vi "nanocal -- nuclear schottky fit V7.vi"() -> ()   [LabVIEW 2021] (continued)
 -> 0.201723581349   ,  \"T\" -> 0.820000000000   ,  \"B\" -> 2.000000000000   ,  \"θ\" -> 0.000000000000   ,  \"Reoff\" -> -1142857.142857141790   ,  \"Imoff\" -> 0.000000000000   ,  \"στ1\" -> 0.016798355334   ,  \"στS\" -> 0.000164505064   ,  \"στN\" -> 0.000022903136    |>   , \n\"IDS0569_220607_RAW_cal__sam_\" ->   <|    \"ζ\" -> 0.000000000000   ,  \"τ1\" -> 0.000000000000   ,  \"τS\" -> 0.000000000000   ,  \"τN\" -> 0.000000000000   ,  \"τC\" -> 0.000000000000   ,  \"κ0\" -> 0.000000000000   ,  \"mm1\" -> 0.000000000000   ,  \"mm2\" -> 0.000000000000   ,  \"mm3\" -> 0.000000000000   ,  \"T\" -> 0.820000000000   ,  \"B\" -> 2.000000000000   ,  \"θ\" -> 0.000000000000   ,  \"Reoff\" -> 0.000000000000   ,  \"Imoff\" -> 0.000000000000   ,  \"στ1\" -> 0.000000000000   ,  \"στS\" -> 0.000000000000   ,  \"στN\" -> 0.000000000000    |>   , \n\"IDS0570_220607_RAW_cal__ref_\" ->   <|    \"ζ\" -> 0.023186603119   ,  \"τ1\" -> 0.069304039551   ,  \"τS\" -> 0.024728755203   ,  \"τN\" -> 0.000615822915   ,  \"τC\" -> 0.002362965503   ,  \"κ0\" -> 0.000000007147   ,  \"mm1\" -> 0.000049060818   ,  \"mm2\" -> 0.027208827859   ,  \"mm3\" -> 0.070341349169   ,  \"T\" -> 1.120000000000   ,  \"B\" -> 2.000000000000   ,  \"θ\" -> 0.000000000000   ,  \"Reoff\" -> -897959.183673471211   ,  \"Imoff\" -> 0.000000000000   ,  \"στ1\" -> 0.007066895477   ,  \"στS\" -> 0.000207495874   ,  \"στN\" -> 0.000024034388    |>   , \n\"IDS0570_220607_RAW_cal__sam_\" ->   <|    \"ζ\" -> 0.000000000000   ,  \"τ1\" -> 0.000000000000   ,  \"τS\" -> 0.000000000000   ,  \"τN\" -> 0.000000000000   ,  \"τC\" -> 0.000000000000   ,  \"κ0\" -> 0.000000000000   ,  \"mm1\" -> 0.000000000000   ,  \"mm2\" -> 0.000000000000   ,  \"mm3\" -> 0.000000000000   ,  \"T\" -> 1.120000000000   ,  \"B\" -> 2.000000000000   ,  \"θ\" -> 0.000000000000   ,  \"Reoff\" -> 0.000000000000   ,  \"Imoff\" -> 0.000000000000   ,  \"στ1\" -> 0.000000000000   ,  \"στS\" -> 0.000000000000   ,  \"στN\" -> 0.000000000000    |>   , \n\"IDS0571_220607_RAW_cal__ref_\" ->   <|    \"ζ\" -> 0.015770363513   ,  \"τ1\" -> 0.071971798635   ,  \"τS\" -> 0.047933574846   ,  \"τN\" -> 0.000365152941   ,  \"τC\" -> 0.002700044906   ,  \"κ0\" -> 0.000000012652   ,  \"mm1\" -> 0.000039747850   ,  \"mm2\" -> 0.050478715429   ,  \"mm3\" -> 0.073213796543   ,  \"T\" -> 1.900000000000   ,  \"B\" -> 2.000000000000   ,  \"θ\" -> 0.000000000000   ,  \"Reoff\" -> -285714.285714287310   ,  \"Imoff\" -> 0.000000000000   ,  \"στ1\" -> 0.006975803229   ,  \"στS\" -> 0.000442024056   ,  \"στN\" -> 0.000016462134    |>   , \n\"IDS0571_220607_RAW_cal__sam_\" ->   <|    \"ζ\" -> 0.000000000000   ,  \"τ1\" -> 0.000000000000   ,  \"τS\" -> 0.000000000000   ,  \"τN\" -> 0.000000000000   ,  \"τC\" -> 0.000000000000   ,  \"κ0\" -> 0.000000000000   ,  \"mm1\" -> 0.000000000000   ,  \"mm2\" -> 0.000000000000   ,  \"mm3\" -> 0.000000000000   ,  \"T\" -> 1.900000000000   ,  \"B\" -> 2.000000000000   ,  \"θ\" -> 0.000000000000   ,  \"Reoff\" -> 0.000000000000   ,  \"Imoff\" -> 0.000000000000   ,  \"στ1\" -> 0.000000000000   ,  \"στS\" -> 0.000000000000   ,  \"στN\" -> 0.000000000000    |>   , \n\"IDS0572_220607_RAW_cal__ref_\" ->   <|    \"ζ\" -> 0.018018584104   ,  \"τ1\" -> 0.047661155544   ,  \"τS\" -> 0.013484677326   ,  \"τN\" -> 0.000256030731   ,  \"τC\" -> 0.002573709531   ,  \"κ0\" -> 0.000000016044   ,  \"mm1\" -> 0.000038452225   ,  \"mm2\" -> 0.016129638273   ,  \"mm3\" -> 0.048055070739   ,  \"T\" -> 2.300000000000   ,  \"B\" -> 2.000000000000   ,  \"θ\" -> 0.000000000000   ,  \"Reoff\" -> -285714.285714287310   ,  \"Imoff\" -> 0.000000000000   ,  \"στ1\" -> 0.009039480993   ,  \"στS\" -> 0.000292801167   ,  \"στN\" -> 0.000013350378    |>   , \n\"IDS0572_220607_RAW_cal__sam_\" ->   <|    \"ζ\" -> 0.000000000000   ,  \"τ1\" -> 0.000000000000   ,  \"τS\" -> 0.000000000000   ,  \"τN\" -> 0.000000000000   ,  \"τC\" -> 0.000000000000   ,  \"κ0\" -> 0.000000000000   ,  \"mm1\" -> 0.000000000000   ,  \"mm2\" -> 0.000000000000   ,  \"mm3\" -> 0.000000000000   ,  \"T\" -> 2.300000000000   ,  \"B\" -> 2.000000000000   ,  \"θ\" -> 0.000000000000   ,  \"Reoff\" -> 0.000000000000   ,  \"Imoff\" -> 0.000000000000   ,  \"στ1\" -> 0.000000000000   ,  \"στS\" -> 0.000000000000   ,  \"στN\" -> 0.000000000000    |>   , \n\"IDS0573_220607_RAW_cal__ref_\" ->   <|    \"ζ\" -> 0.017854709230   ,  \"τ1\" -> 0.048990500372   ,  \"τS\" -> 0.009409191095   ,  \"τN\" -> 0.000133052666   ,  \"τC\" -> 0.002613702785   ,  \"κ0\" -> 0.000000022548   ,  \"mm1\" -> 0.000036125485   ,  \"mm2\" -> 0.012110331944   ,  \"mm3\" -> 0.049170363477   ,  \"T\" -> 3.100000000000   ,  \"B\" -> 2.000000000000   ,  \"θ\" -> 0.000000000000   ,  \"Reoff\" -> -163265.306122448295   ,  \"Imoff\" -> 0.000000000000   ,  \"στ1\" -> 0.003929388168   ,  \"στS\" -> 0.000082158552   ,  \"στN\" -> 0.000004662808    |>   , \n\"IDS0573_220607_RAW_cal__sam_\" ->   <|    \"ζ\" -> 0.000000000000   ,  \"τ1\" -> 0.000000000000   ,  \"τS\" -> 0.000000000000   ,  \"τN\" -> 0.000000000000   ,  \"τC\" -> 0.000000000000   ,  \"κ0\" -> 0.000000000000   ,  \"mm1\" -> 0.000000000000   ,  \"mm2\" -> 0.000000000000   ,  \"mm3\" -> 0.000000000000   ,  \"T\" -> 3.100000000000   ,  \"B\" -> 2.000000000000   ,  \"θ\" -> 0.000000000000   ,  \"Reoff\" -> 0.000000000000   ,  \"Imoff\" -> 0.000000000000   ,  \"στ1\" -> 0.000000000000   ,  \"στS\" -> 0.000000000000   ,  \"στN\" -> 0.000000000000    |>   , \n\"IDS0574_220607_RAW_cal__ref_\" ->   <|    \"ζ\" -> 0.021296069589   ,  \"τ1\" -> 0.048193111718   ,  \"τS\" -> 0.005769221839   ,  \"τN\" -> 0.000085869671   ,  \"τC\" -> 0.001966024103   ,  \"κ0\" -> 0.000000055540   ,  \"mm1\" -> 0.000030859965   ,  \"mm2\" -> 0.007810308294   ,  \"mm3\" -> 0.048297749508   ,  \"T\" -> 5.700000000000   ,  \"B\" -> 2.000000000000   ,  \"θ\" -> 0.000000000000   ,  \"Reoff\" -> -89795.918367346749   ,  \"Imoff\" -> 0.000000000000   ,  \"στ1\" -> 0.003900504752   ,  \"στS\" -> 0.000042384921   ,  \"στN\" -> 0.000002866550    |>   , \n\"IDS0574_220607_RAW_cal__sam_\" ->   <|    \"ζ\" -> 0.000000000000   ,  \"τ1\" -> 0.000000000000   ,  \"τS\" -> 0.000000000000   ,  \"τN\" -> 0.000000000000   ,  \"τC\" -> 0.000000000000   ,  \"κ0\" -> 0.000000000000   ,  \"mm1\" -> 0.000000000000   ,  \"mm2\" -> 0.000000000000   ,  \"mm3\" -> 0.000000000000   ,  \"T\" -> 5.700000000000   ,  \"B\" -> 2.000000000000   ,  \"θ\" -> 0.000000000000   ,  \"Reoff\" -> 0.000000000000   ,  \"Imoff\" -> 0.000000000000   ,  \"στ1\" -> 0.000000000000   ,  \"στS\" -> 0.000000000000   ,  \"στN\" -> 0.000000000000    |>   , \n\"IDS0578_220608_RAW_cal__ref_\" ->   <|    \"ζ\" -> 0.260580240331   ,  \"τ1\" -> 0.233392220968   ,  \"τS\" -> 0.019337528339   ,  \"τN\" -> 0.006746984129   ,  \"τC\" -> 0.000809912718   ,  \"κ0\" -> 0.000000000898   ,  \"mm1\" -> 0.000163092082   ,  \"mm2\" -> 0.024046559857   ,  \"mm3\" -> 0.242874102744   ,  \"T\" -> 0.200000000000   ,  \"B\" -> 2.000000000000   ,  \"θ\" -> 90.000000000000   ,  \"Reoff\" -> -51020408.163265287900   ,  \"Imoff\" -> 0.000000000000   ,  \"στ1\" -> 0.360874017703   ,  \"στS\" -> 0.000459944418   ,  \"στN\" -> 0.007141056200    |>   , \n\"IDS0578_220608_RAW_cal__sam_\" ->   <|    \"ζ\" -> 0.000000000000   ,  \"τ1\" -> 0.000000000000   ,  \"τS\" -> 0.000000000000   ,  \"τN\" -> 0.000000000000   ,  \"τC\" -> 0.000000000000   ,  \"κ0\" -> 0.000000000000   ,  \"mm1\" -> 0.000000000000   ,  \"mm2\" -> 0.000000000000   ,  \"mm3\" -> 0.000000000000   ,  \"T\" -> 0.200000000000   ,  \"B\" -> 2.000000000000   ,  \"θ\" -> 90.000000000000   ,  \"Reoff\" -> 0.000000000000   ,  \"Imoff\" -> 0.000000000000   ,  \"στ1\" -> 0.000000000000   ,  \"στS\" -> 0.000000000000   ,  \"στN\" -> 0.000000000000    |>   , \n\"IDS0579_220608_RAW_cal__ref_\" ->   <|    \"ζ\" -> 0.358041732305   ,  \"τ1\" -> 0.218984893341   ,  \"τS\" -> 0.022109893709   ,  \"τN\" -> 0.011578421119   ,  \"τC\" -> 0.000774433851   ,  \"κ0\" -> 0.000000000705   ,  \"mm1\" -> 0.000200343737   ,  \"mm2\" -> 0.028269791705   ,  \"mm3\" -> 0.237039329177   ,  \"T\" -> 0.170000000000   ,  \"B\" -> 2.000000000000   ,  \"θ\" -> 90.000000000000   ,  \"Reoff\" -> -83673469.387755096000   ,  \"Imoff\" -> 0.000000000000   ,  \"στ1\" -> 0.324633037067   ,  \"στS\" -> 0.000730773074   ,  \"στN\" -> 0.013143956795    |>   , \n\"IDS0579_220608_RAW_cal__sam_\" ->   <|    \"ζ\" -> 0.000000000000   ,  \"τ1\" -> 0.000000000000   ,  \"τS\" -> 0.000000000000   ,  \"τN\" -> 0.000000000000   ,  \"τC\" -> 0.000000000000   ,  \"κ0\" -> 0.000000000000   ,  \"mm1\" -> 0.000000000000   ,  \"mm2\" -> 0.000000000000   ,  \"mm3\" -> 0.000000000000   ,  \"T\" -> 0.170000000000   ,  \"B\" -> 2.000000000000   ,  \"θ\" -> 90.000000000000   ,  \"Reoff\" -> 0.000000000000   ,  \"Imoff\" -> 0.000000000000   ,  \"στ1\" -> 0.000000000000   ,  \"στS\" -> 0.000000000000   ,  \"στN\" -> 0.000000000000    |>   , \n\"IDS0580_220608_RAW_cal__ref_\" ->   <|    \"ζ\" -> 0.444194308226   ,  \"τ1\" -> 0.247703542844   ,  \"τS\" -> 0.025021615076   ,  \"τN\" -> 0.015371954390   ,  \"τC\" -> 0.000794757601   ,  \"κ0\" -> 0.000000000600   ,  \"mm1\" -> 0.000240752300   ,  \"mm2\" -> 0.033248610212   ,  \"mm3\" -> 0.273345101045   ,  \"T\" -> 0.150000000000   ,  \"B\" -> 2.000000000000   ,  \"θ\" -> 90.000000000000   ,  \"Reoff\" -> -104081632.653061211000   ,  \"Imoff\" -> 0.000000000000   ,  \"στ1\" -> 0.811876218659   ,  \"στS\" -> 0.001521304973   ,  \"στN\" -> 0.040822562310    |>   , \n\"IDS0580_220608_RAW_cal__sam_\" ->   <|    \"ζ\" -> 0.000000000000   ,  \"τ1\" -> 0.000000000000   ,  \"τS\" -> 0.000000000000   ,  \"τN\" -> 0.000000000000   ,  \"τC\" -> 0.000000000000   ,  \"κ0\" -> 0.000000000000   ,  \"mm1\" -> 0.000000000000   ,  \"mm2\" -> 0.000000000000   ,  \"mm3\" -> 0.000000000000   ,  \"T\" -> 0.150000000000   ,  \"B\" -> 2.000000000000   ,  \"θ\" -> 90.000000000000   ,  \"Reoff\" -> 0.000000000000   ,  \"Imoff\" -> 0.000000000000   ,  \"στ1\" -> 0.000000000000   ,  \"στS\" -> 0.000000000000   ,  \"στN\" -> 0.000000000000    |>   , \n\"IDS0581_220608_RAW_cal__ref_\" ->   <|    \"ζ\" -> 0.686806962981   ,  \"τ1\" -> 0.191964510357   ,  \"τS\" -> 0.031477597051   ,  \"τN\" -> 0.029789944795   ,  \"τC\" -> 0.000797477821   ,  \"κ0\" -> 0.000000000433   ,  \"mm1\" -> 0.000321816656   ,  \"mm2\" -> 0.040244297441   ,  \"mm3\" -> 0.255542390272   ,  \"T\" -> 0.120000000000   ,  \"B\" -> 2.000000000000   ,  \"θ\" -> 90.000000000000   ,  \"Reoff\" -> -218367346.938775510000   ,  \"Imoff\" -> 0.000000000000   ,  \"στ1\" -> 0.248597488998   ,  \"στS\" -> 0.002831181242   ,  \"στN\" -> 0.031806706752    |>   , \n\"IDS0581_220608_RAW_cal__sam_\" ->   <|    \"ζ\" -> 0.000000000000   ,  \"τ1\" -> 0.000000000000   ,  \"τS\" -> 0.000000000000   ,  \"τN\" -> 0.000000000000   ,  \"τC\" -> 0.000000000000   ,  \"κ0\" -> 0.000000000000   ,  \"mm1\" -> 0.000000000000   ,  \"mm2\" -> 0.000000000000   ,  \"mm3\" -> 0.000000000000   ,  \"T\" -> 0.120000000000   ,  \"B\" -> 2.000000000000   ,  \"θ\" -> 90.000000000000   ,  \"Reoff\" -> 0.000000000000   ,  \"Imoff\" -> 0.000000000000   ,  \"στ1\" -> 0.000000000000   ,  \"στS\" -> 0.000000000000   ,  \"στN\" -> 0.000000000000    |>   , \n\"IDS0582_220608_RAW_cal__ref_\" ->   <|    \"ζ\" -> 0.166369563634   ,  \"τ1\" -> 0.241506341921   ,  \"τS\" -> 0.016551953229   ,  \"τN\" -> 0.004476656392   ,  \"τC\" -> 0.000955255274   ,  \"κ0\" -> 0.000000001230   ,  \"mm1\" -> 0.000130674320   ,  \"mm2\" -> 0.019667491815   ,  \"mm3\" -> 0.247190561287   ,  \"T\" -> 0.250000000000   ,  \"B\" -> 2.000000000000   ,  \"θ\" -> 90.000000000000   ,  \"Reoff\" -> -23265306.122448980800   ,  \"Imoff\" -> 0.000000000000   ,  \"στ1\" -> 0.210252832674   ,  \"στS\" -> 0.000349343663   ,  \"στN\" -> 0.005793752107    |>   , \n\"IDS0582_220608_RAW_cal__sam_\" ->   <|    \"ζ\" -> 0.000000000000   ,  \"τ1\" -> 0.000000000000   ,  \"τS\" -> 0.000000000000   ,  \"τN\" -> 0.000000000000   ,  \"τC\" -> 0.000000000000   ,  \"κ0\" -> 0.000000000000   ,  \"mm1\" -> 0.000000000000   ,  \"mm2\" -> 0.000000000000   ,  \"mm3\" -> 0.000000000000   ,  \"T\" -> 0.250000000000   ,  \"B\" -> 2.000000000000   ,  \"θ\" -> 90.000000000000   ,  \"Reoff\" -> 0.000000000000   ,  \"Imoff\" -> 0.000000000000   ,  \"στ1\" -> 0.000000000000   ,  \"στS\" -> 0.000000000000   ,  \"στN\" -> 0.000000000000    |>   , \n\"IDS0583_220608_RAW_cal__ref_\" ->   <|    \"ζ\" -> 0.118361182005   ,  \"τ1\" -> 0.150636490656   ,  \"τS\" -> 0.015529851966   ,  \"τN\" -> 0.003531374182   ,  \"τC\" -> 0.001007690492   ,  \"κ0\" -> 0.000000001529   ,  \"mm1\" -> 0.000101358307   ,  \"mm2\" -> 0.017747047219   ,  \"mm3\" -> 0.155113111027   ,  \"T\" -> 0.300000000000   ,  \"B\" -> 2.000000000000   ,  \"θ\" -> 90.000000000000   ,  \"Reoff\" -> -15102040.816326528800   ,  \"Imoff\" -> 0.000000000000   ,  \"στ1\" -> 0.078929426255   ,  \"στS\" -> 0.000167827635   ,  \"στN\" -> 0.002346663512    |>   , \n\"IDS0583_220608_RAW_cal__sam_\" ->   <|    \"ζ\" -> 0.000000000000   ,  \"τ1\" -> 0.000000000000   ,  \"τS\" -> 0.000000000000   ,  \"τN\" -> 0.000000000000   ,  \"τC\" -> 0.000000000000   ,  \"κ0\" -> 0.000000000000   ,  \"mm1\" -> 0.000000000000   ,  \"mm2\" -> 0.000000000000   ,  \"mm3\" -> 0.000000000000   ,  \"T\" -> 0.300000000000   ,  \"B\" -> 2.000000000000   ,  \"θ\" -> 90.000000000000   ,  \"Reoff\" -> 0.000000000000   ,  \"Imoff\" -> 0.000000000000   ,  \"στ1\" -> 0.000000000000   ,  \"στS\" -> 0.000000000000   ,  \"στN\" -> 0.000000000000    |>   , \n\"IDS0584_220608_RAW_cal__ref_\" ->   <|    \"ζ\" -> 0.085716797729   ,  \"τ1\" -> 0.145541921942   ,  \"τS\" -> 0.014790459938   ,  \"τN\" -> 0.003022723579   ,  \"τC\" -> 0.001204929117   ,  \"κ0\" -> 0.000000001932   ,  \"mm1\" -> 0.000088946369   ,  \"mm2\" -> 0.016747642578   ,  \"mm3\" -> 0.149250334678   ,  \"T\" -> 0.360000000000   ,  \"B\" -> 2.000000000000   ,  \"θ\" -> 90.000000000000   ,  \"Reoff\" -> -8571428.571428582080   ,  \"Imoff\" -> 0.000000000000   ,  \"στ1\" -> 0.049017314235   ,  \"στS\" -> 0.000077215540   ,  \"στN\" -> 0.000273627633    |>   , \n\"IDS0584_220608_RAW_cal__sam_\" ->   <|    \"ζ\" -> 0.000000000000   ,  \"τ1\" -> 0.000000000000   ,  \"τS\" -> 0.000000000000   ,  \"τN\" -> 0.000000000000   ,  \"τC\" -> 0.000000000000   ,  \"κ0\" -> 0.000000000000   ,  \"mm1\" -> 0.000000000000   ,  \"mm2\" -> 0.000000000000   ,  \"mm3\" -> 0.000000000000   ,  \"T\" -> 0.360000000000   ,  \"B\" -> 2.000000000000   ,  \"θ\" -> 90.000000000000   ,  \"Reoff\" -> 0.000000000000   ,  \"Imoff\" -> 0.000000000000   ,  \"στ1\" -> 0.000000000000   ,  \"στS\" -> 0.000000000000   ,  \"στN\" -> 0.000000000000    |>   , \n\"IDS0585_220608_RAW_cal__ref_\" ->   <|    \"ζ\" -> 0.064153972834   ,  \"τ1\" -> 0.145990399088   ,  \"τS\" -> 0.014755700071   ,  \"τN\" -> 0.002470459255   ,  \"τC\" -> 0.001390626850   ,  \"κ0\" -> 0.000000002341   ,  \"mm1\" -> 0.000077364865   ,  \"mm2\" -> 0.016676693112   ,  \"mm3\" -> 0.148958253844   ,  \"T\" -> 0.420000000000   ,  \"B\" -> 2.000000000000   ,  \"θ\" -> 90.000000000000   ,  \"Reoff\" -> -4530612.244897958820   ,  \"Imoff\" -> 0.000000000000   ,  \"στ1\" -> 0.010117026609   ,  \"στS\" -> 0.000141538965   ,  \"στN\" -> 0.000077781764    |>   , \n\"IDS0585_220608_RAW_cal__sam_\" ->   <|    \"ζ\" -> 0.000000000000   ,  \"τ1\" -> 0.000000000000   ,  \"τS\" -> 0.000000000000   ,  \"τN\" -> 0.000000000000   ,  \"τC\" -> 0.000000000000   ,  \"κ0\" -> 0.000000000000   ,  \"mm1\" -> 0.000000000000   ,  \"mm2\" -> 0.000000000000   ,  \"mm3\" -> 0.000000000000   ,  \"T\" -> 0.420000000000   ,  \"B\" -> 2.000000000000   ,  \"θ\" -> 90.000000000000   ,  \"Reoff\" -> 0.000000000000   ,  \"Imoff\" -> 0.000000000000   ,  \"στ1\" -> 0.000000000000   ,  \"στS\" -> 0.000000000000   ,  \"στN\" -> 0.000000000000    |>   , \n\"IDS0586_220608_RAW_cal__ref_\" ->   <|    \"ζ\" -> 0.050400440296   ,  \"τ1\" -> 0.120007371635   ,  \"τS\" -> 0.015618683096   ,  \"τN\" -> 0.001956039129   ,  \"τC\" -> 0.001501517777   ,  \"κ0\" -> 0.000000002996   ,  \"mm1\" -> 0.000066249745   ,  \"mm2\" -> 0.017490709551   ,  \"mm3\" -> 0.122412426079   ,  \"T\" -> 0.520000000000   ,  \"B\" -> 2.000000000000   ,  \"θ\" -> 90.000000000000   ,  \"Reoff\" -> -3877551.020408162850   ,  \"Imoff\" -> 0.000000000000   ,  \"στ1\" -> 0.009823024060   ,  \"στS\" -> 0.000148546431   ,  \"στN\" -> 0.000049706708    |>   , \n\"IDS0586_220608_RAW_cal__sam_\" ->   <|    \"ζ\" -> 0.000000000000   ,  \"τ1\" -> 0.000000000000   ,  \"τS\" -> 0.000000000000   ,  \"τN\" -> 0.000000000000   ,  \"τC\" -> 0.000000000000   ,  \"κ0\" -> 0.000000000000   ,  \"mm1\" -> 0.000000000000   ,  \"mm2\" -> 0.000000000000   ,  \"mm3\" -> 0.000000000000   ,  \"T\" -> 0.520000000000   ,  \"B\" -> 2.000000000000   ,  \"θ\" -> 90.000000000000   ,  \"Reoff\" -> 0.000000000000   ,  \"Imoff\" -> 0.000000000000   ,  \"στ1\" -> 0.000000000000   ,  \"στS\" -> 0.000000000000   ,  \"στN\" -> 0.000000000000    |>   , \n\"IDS0587_220608_RAW_cal__ref_\" ->   <|    \"ζ\" -> 0.040966221247   ,  \"τ1\" -> 0.107264057054   ,  \"τS\" -> 0.017218763514   ,  \"τN\" -> 0.001743151532   ,  \"τC\" -> 0.001685988856   ,  \"κ0\" -> 0.000000003666   ,  \"mm1\" -> 0.000060834390   ,  \"mm2\" -> 0.019154933369   ,  \"mm3\" -> 0.109472991205   ,  \"T\" -> 0.620000000000   ,  \"B\" -> 2.000000000000   ,  \"θ\" -> 90.000000000000   ,  \"Reoff\" -> -2816326.530612244270   ,  \"Imoff\" -> 0.000000000000   ,  \"στ1\" -> 0.008843102756   ,  \"στS\" -> 0.000179440929   ,  \"στN\" -> 0.000073166949    |>   , \n\"IDS0587_220608_RAW_cal__sam_\" ->   <|    \"ζ\" -> 0.000000000000   ,  \"τ1\" -> 0.000000000000   ,  \"τS\" -> 0.000000000000   ,  \"τN\" -> 0.000000000000   ,  \"τC\" -> 0.000000000000   ,  \"κ0\" -> 0.000000000000   ,  \"mm1\" -> 0.000000000000   ,  \"mm2\" -> 0.000000000000   ,  \"mm3\" -> 0.000000000000   ,  \"T\" -> 0.620000000000   ,  \"B\" -> 2.000000000000   ,  \"θ\" -> 90.000000000000   ,  \"Reoff\" -> 0.000000000000   ,  \"Imoff\" -> 0.000000000000   ,  \"στ1\" -> 0.000000000000   ,  \"στS\" -> 0.000000000000   ,  \"στN\" -> 0.000000000000    |>   , \n\"IDS0588_220608_RAW_cal__ref_\" ->   <|    \"ζ\" -> 0.027966572573   ,  \"τ1\" -> 0.110878949003   ,  \"τS\" -> 0.020906801035   ,  \"τN\" -> 0.001317162593   ,  \"τC\" -> 0.002396852626   ,  \"κ0\" -> 0.000000005050   ,  \"mm1\" -> 0.000058809998   ,  \"mm2\" -> 0.023466150465   ,  \"mm3\" -> 0.112596332885   ,  \"T\" -> 0.820000000000   ,  \"B\" -> 2.000000000000   ,  \"θ\" -> 90.000000000000   ,  \"Reoff\" -> -1020408.163265304640   ,  \"Imoff\" -> 0.000000000000   ,  \"στ1\" -> 0.009326447287   ,  \"στS\" -> 0.000184300760   ,  \"στN\" -> 0.000049241490    |>   , \n\"IDS0588_220608_RAW_cal__sam_\" ->   <|    \"ζ\" -> 0.000000000000   ,  \"τ1\" -> 0.000000000000   ,  \"τS\" -> 0.000000000000   ,  \"τN\" -> 0.000000000000   ,  \"τC\" -> 0.000000000000   ,  \"κ0\" -> 0.000000000000   ,  \"mm1\" -> 0.000000000000   ,  \"mm2\" -> 0.000000000000   ,  \"mm3\" -> 0.000000000000   ,  \"T\" -> 0.820000000000   ,  \"B\" -> 2.000000000000   ,  \"θ\" -> 90.000000000000   ,  \"Reoff\" -> 0.000000000000   ,  \"Imoff\" -> 0.000000000000   ,  \"στ1\" -> 0.000000000000   ,  \"στS\" -> 0.000000000000   ,  \"στN\" -> 0.000000000000    |>   , \n\"IDS0589_220608_RAW_cal__ref_\" ->   <|    \"ζ\" -> 0.023281533249   ,  \"τ1\" -> 0.113795019123   ,  \"τS\" -> 0.028800719763   ,  \"τN\" -> 0.000699230708   ,  \"τC\" -> 0.002435159498   ,  \"κ0\" -> 0.000000007137   ,  \"mm1\" -> 0.000051258085   ,  \"mm2\" -> 0.031580340212   ,  \"mm3\" -> 0.114785334873   ,  \"T\" -> 1.120000000000   ,  \"B\" -> 2.000000000000   ,  \"θ\" -> 90.000000000000   ,  \"Reoff\" -> -938775.510204080491   ,  \"Imoff\" -> 0.000000000000   ,  \"στ1\" -> 0.007362854909   ,  \"στS\" -> 0.000278698493   ,  \"στN\" -> 0.000011047668    |>   , \n\"IDS0589_220608_RAW_cal__sam_\" ->   <|    \"ζ\" -> 0.000000000000   ,  \"τ1\" -> 0.000000000000   ,  \"τS\" -> 0.000000000000   ,  \"τN\" -> 0.000000000000   ,  \"τC\" -> 0.000000000000   ,  \"κ0\" -> 0.000000000000   ,  \"mm1\" -> 0.000000000000   ,  \"mm2\" -> 0.000000000000   ,  \"mm3\" -> 0.000000000000   ,  \"T\" -> 1.120000000000   ,  \"B\" -> 2.000000000000   ,  \"θ\" -> 90.000000000000   ,  \"Reoff\" -> 0.000000000000   ,  \"Imoff\" -> 0.000000000000   ,  \"στ1\" -> 0.000000000000   ,  \"στS\" -> 0.000000000000   ,  \"στN\" -> 0.000000000000    |>   , \n\"IDS0590_220608_RAW_cal__ref_\" ->   <|    \"ζ\" -> 0.017825574653   ,  \"τ1\" -> 0.116468007826   ,  \"τS\" -> 0.043141778106   ,  \"τN\" -> 0.000373800852   ,  \"τC\" -> 0.002722368928   ,  \"κ0\" -> 0.000000010436   ,  \"mm1\" -> 0.000044937841   ,  \"mm2\" -> 0.046336871767   ,  \"mm3\" -> 0.117099836305   ,  \"T\" -> 1.600000000000   ,  \"B\" -> 2.000000000000   ,  \"θ\" -> 90.000000000000   ,  \"Reoff\" -> -510204.081632653076   ,  \"Imoff\" -> 0.000000000000   ,  \"στ1\" -> 0.011139723010   ,  \"στS\" -> 0.000337999811   ,  \"στN\" -> 0.000011692762    |>   , \n\"IDS0590_220608_RAW_cal__sam_\" ->   <|    \"ζ\" -> 0.000000000000   ,  \"τ1\" -> 0.000000000000   ,  \"τS\" -> 0.000000000000   ,  \"τN\" -> 0.000000000000   ,  \"τC\" -> 0.000000000000   ,  \"κ0\" -> 0.000000000000   ,  \"mm1\" -> 0.000000000000   ,  \"mm2\" -> 0.000000000000   ,  \"mm3\" -> 0.000000000000   ,  \"T\" -> 1.600000000000   ,  \"B\" -> 2.000000000000   ,  \"θ\" -> 90.000000000000   ,  \"Reoff\" -> 0.000000000000   ,  \"Imoff\" -> 0.000000000000   ,  \"στ1\" -> 0.000000000000   ,  \"στS\" -> 0.000000000000   ,  \"στN\" -> 0.000000000000    |>   , \n\"IDS0591_220608_RAW_cal__ref_\" ->   <|    \"ζ\" -> 0.018966449660   ,  \"τ1\" -> 0.110092167291   ,  \"τS\" -> 0.012256930668   ,  \"τN\" -> 0.000242942358   ,  \"τC\" -> 0.002442548821   ,  \"κ0\" -> 0.000000015655   ,  \"mm1\" -> 0.000038124511   ,  \"mm2\" -> 0.014855231202   ,  \"mm3\" -> 0.110378311637   ,  \"T\" -> 2.300000000000   ,  \"B\" -> 2.000000000000   ,  \"θ\" -> 90.000000000000   ,  \"Reoff\" -> -330612.244897959171   ,  \"Imoff\" -> 0.000000000000   ,  \"στ1\" -> 0.010082943855   ,  \"στS\" -> 0.000135571063   ,  \"στN\" -> 0.000004812408    |>   , \n\"IDS0591_220608_RAW_cal__sam_\" ->   <|    \"ζ\" -> 0.000000000000   ,  \"τ1\" -> 0.000000000000   ,  \"τS\" -> 0.000000000000   ,  \"τN\" -> 0.000000000000   ,  \"τC\" -> 0.000000000000   ,  \"κ0\" -> 0.000000000000   ,  \"mm1\" -> 0.000000000000   ,  \"mm2\" -> 0.000000000000   ,  \"mm3\" -> 0.000000000000   ,  \"T\" -> 2.300000000000   ,  \"B\" -> 2.000000000000   ,  \"θ\" -> 90.000000000000   ,  \"Reoff\" -> 0.000000000000   ,  \"Imoff\" -> 0.000000000000   ,  \"στ1\" -> 0.000000000000   ,  \"στS\" -> 0.000000000000   ,  \"στN\" -> 0.000000000000    |>   , \n\"IDS0592_220608_RAW_cal__ref_\" ->   <|    \"ζ\" -> 0.019357316755   ,  \"τ1\" -> 0.109232590741   ,  \"τS\" -> 0.009736709939   ,  \"τN\" -> 0.000148850192   ,  \"τC\" -> 0.002349823712   ,  \"κ0\" -> 0.000000022430   ,  \"mm1\" -> 0.000036187001   ,  \"mm2\" -> 0.012219724348   ,  \"mm3\" -> 0.109403421154   ,  \"T\" -> 3.100000000000   ,  \"B\" -> 2.000000000000   ,  \"θ\" -> 90.000000000000   ,  \"Reoff\" -> -232653.061224489822   ,  \"Imoff\" -> 0.000000000000   ,  \"στ1\" -> 0.008987310328   ,  \"στS\" -> 0.000109754464   ,  \"στN\" -> 0.000004448461    |>   , \n\"IDS0592_220608_RAW_cal__sam_\" ->   <|    \"ζ\" -> 0.000000000000   ,  \"τ1\" -> 0.000000000000   ,  \"τS\" -> 0.000000000000   ,  \"τN\" -> 0.000000000000   ,  \"τC\" -> 0.000000000000   ,  \"κ0\" -> 0.000000000000   ,  \"mm1\" -> 0.000000000000   ,  \"mm2\" -> 0.000000000000   ,  \"mm3\" -> 0.000000000000   ,  \"T\" -> 3.100000000000   ,  \"B\" -> 2.000000000000   ,  \"θ\" -> 90.000000000000   ,  \"Reoff\" -> 0.000000000000   ,  \"Imoff\" -> 0.000000000000   ,  \"στ1\" -> 0.000000000000   ,  \"στS\" -> 0.000000000000   ,  \"στN\" -> 0.000000000000    |>   , \n\"IDS0593_220608_RAW_cal__ref_\" ->   <|    \"ζ\" -> 0.022440001502   ,  \"τ1\" -> 0.108774382212   ,  \"τS\" -> 0.005986162529   ,  \"τN\" -> 0.000081229667   ,  \"τC\" -> 0.001771054543   ,  \"κ0\" -> 0.000000055356   ,  \"mm1\" -> 0.000030262826   ,  \"mm2\" -> 0.007854826642   ,  \"mm3\" -> 0.108863891772   ,  \"T\" -> 5.700000000000   ,  \"B\" -> 2.000000000000   ,  \"θ\" -> 90.000000000000   ,  \"Reoff\" -> -118367.346938775503   ,  \"Imoff\" -> 0.000000000000   ,  \"στ1\" -> 0.009498599420   ,  \"στS\" -> 0.000059156113   ,  \"στN\" -> 0.000001864029    |>   , \n\"IDS0593_220608_RAW_cal__sam_\" ->   <|    \"ζ\" -> 0.000000000000   ,  \"τ1\" -> 0.000000000000   ,  \"τS\" -> 0.000000000000   ,  \"τN\" -> 0.000000000000   ,  \"τC\" -> 0.000000000000   ,  \"κ0\" -> 0.000000000000   ,  \"mm1\" -> 0.000000000000   ,  \"mm2\" -> 0.000000000000   ,  \"mm3\" -> 0.000000000000   ,  \"T\" -> 5.700000000000   ,  \"B\" -> 2.000000000000   ,  \"θ\" -> 90.000000000000   ,  \"Reoff\" -> 0.000000000000   ,  \"Imoff\" -> 0.000000000000   ,  \"στ1\" -> 0.000000000000   ,  \"στS\" -> 0.000000000000   ,  \"στN\" -> 0.000000000000    |>   , \n\"IDS0595_220608_RAW_cal__ref_\" ->   <|    \"ζ\" -> 0.258873400405   ,  \"τ1\" -> 0.044703065528   ,  \"τS\" -> 0.045959272173   ,  \"τN\" -> 0.010257269472   ,  \"τC\" -> 0.000790030370   ,  \"κ0\" -> 0.000000000876   ,  \"mm1\" -> 0.000160711520   ,  \"mm2\" -> 0.030566838015   ,  \"mm3\" -> 0.085535055303   ,  \"T\" -> 0.200000000000   ,  \"B\" -> 4.000000000000   ,  \"θ\" -> 90.000000000000   ,  \"Reoff\" -> -50122448.979591846500   ,  \"Imoff\" -> 0.000000000000   ,  \"στ1\" -> 0.022832091218   ,  \"στS\" -> 0.001836443517   ,  \"στN\" -> 0.003113362841    |>   , \n\"IDS0595_220608_RAW_cal__sam_\" ->   <|    \"ζ\" -> 0.000000000000   ,  \"τ1\" -> 0.000000000000   ,  \"τS\" -> 0.000000000000   ,  \"τN\" -> 0.000000000000   ,  \"τC\" -> 0.000000000000   ,  \"κ0\" -> 0.000000000000   ,  \"mm1\" -> 0.000000000000   ,  \"mm2\" -> 0.000000000000   ,  \"mm3\" -> 0.000000000000   ,  \"T\" -> 0.200000000000   ,  \"B\" -> 4.000000000000   ,  \"θ\" -> 90.000000000000   ,  \"Reoff\" -> 0.000000000000   ,  \"Imoff\" -> 0.000000000000   ,  \"στ1\" -> 0.000000000000   ,  \"στS\" -> 0.000000000000   ,  \"στN\" -> 0.000000000000    |>   , \n\"IDS0596_220608_RAW_cal__ref_\" ->   <|    \"ζ\" -> 0.360293553844   ,  \"τ1\" -> 0.054491247205   ,  \"τS\" -> 0.052365925569   ,  \"τN\" -> 0.021163604976   ,  \"τC\" -> 0.000735569124   ,  \"κ0\" -> 0.000000000708   ,  \"mm1\" -> 0.000193352298   ,  \"mm2\" -> 0.031708785760   ,  \"mm3\" -> 0.123346424689   ,  \"T\" -> 0.170000000000   ,  \"B\" -> 4.000000000000   ,  \"θ\" -> 90.000000000000   ,  \"Reoff\" -> -91020408.163265347500   ,  \"Imoff\" -> 0.000000000000   ,  \"στ1\" -> 0.039757626567   ,  \"στS\" -> 0.004569334706   ,  \"στN\" -> 0.007867287880    |>   , \n\"IDS0596_220608_RAW_cal__sam_\" ->   <|    \"ζ\" -> 0.000000000000   ,  \"τ1\" -> 0.000000000000   ,  \"τS\" -> 0.000000000000   ,  \"τN\" -> 0.000000000000   ,  \"τC\" -> 0.000000000000   ,  \"κ0\" -> 0.000000000000   ,  \"mm1\" -> 0.000000000000   ,  \"mm2\" -> 0.000000000000   ,  \"mm3\" -> 0.000000000000   ,  \"T\" -> 0.170000000000   ,  \"B\" -> 4.000000000000   ,  \"θ\" -> 90.000000000000   ,  \"Reoff\" -> 0.000000000000   ,  \"Imoff\" -> 0.000000000000   ,  \"στ1\" -> 0.000000000000   ,  \"στS\" -> 0.000000000000   ,  \"στN\" -> 0.000000000000    |>   , \n\"IDS0597_220608_RAW_cal__ref_\" ->   <|    \"ζ\" -> 0.463165977160   ,  \"τ1\" -> 0.056305688672   ,  \"τS\" -> 0.058936067293   ,  \"τN\" -> 0.032266294348   ,  \"τC\" -> 0.000690215533   ,  \"κ0\" -> 0.000000000590   ,  \"mm1\" -> 0.000217293879   ,  \"mm2\" -> 0.030581784486   ,  \"mm3\" -> 0.159641018430   ,  \"T\" -> 0.150000000000   ,  \"B\" -> 4.000000000000   ,  \"θ\" -> 90.000000000000   ,  \"Reoff\" -> -129873469.387755096000   ,  \"Imoff\" -> 0.000000000000   ,  \"στ1\" -> 0.023207253822   ,  \"στS\" -> 0.004087293472   ,  \"στN\" -> 0.007020371426    |>   , \n\"IDS0597_220608_RAW_cal__sam_\" ->   <|    \"ζ\" -> 0.000000000000   ,  \"τ1\" -> 0.000000000000   ,  \"τS\" -> 0.000000000000   ,  \"τN\" -> 0.000000000000   ,  \"τC\" -> 0.000000000000   ,  \"κ0\" -> 0.000000000000   ,  \"mm1\" -> 0.000000000000   ,  \"mm2\" -> 0.000000000000   ,  \"mm3\" -> 0.000000000000   ,  \"T\" -> 0.150000000000   ,  \"B\" -> 4.000000000000   ,  \"θ\" -> 90.000000000000   ,  \"Reoff\" -> 0.000000000000   ,  \"Imoff\" -> 0.000000000000   ,  \"στ1\" -> 0.000000000000   ,  \"στS\" -> 0.000000000000   ,  \"στN\" -> 0.000000000000    |>   , \n\"IDS0598_220609_RAW_cal__ref_\" ->   <|    \"ζ\" -> 0.667698633058   ,  \"τ1\" -> 0.058414013789   ,  \"τS\" -> 0.079345994200   ,  \"τN\" -> 0.070623883647   ,  \"τC\" -> 0.000796244293   ,  \"κ0\" -> 0.000000000447   ,  \"mm1\" -> 0.000317638863   ,  \"mm2\" -> 0.027565245662   ,  \"mm3\" -> 0.281431933842   ,  \"T\" -> 0.120000000000   ,  \"B\" -> 4.000000000000   ,  \"θ\" -> 90.000000000000   ,  \"Reoff\" -> -199400000.000000000000   ,  \"Imoff\" -> 0.000000000000   ,  \"στ1\" -> 0.061256230703   ,  \"στS\" -> 0.021100595545   ,  \"στN\" -> 0.037759623008    |>   , \n\"IDS0598_220609_RAW_cal__sam_\" ->   <|    \"ζ\" -> 0.000000000000   ,  \"τ1\" -> 0.000000000000   ,  \"τS\" -> 0.000000000000   ,  \"τN\" -> 0.000000000000   ,  \"τC\" -> 0.000000000000   ,  \"κ0\" -> 0.000000000000   ,  \"mm1\" -> 0.000000000000   ,  \"mm2\" -> 0.000000000000   ,  \"mm3\" -> 0.000000000000   ,  \"T\" -> 0.120000000000   ,  \"B\" -> 4.000000000000   ,  \"θ\" -> 90.000000000000   ,  \"Reoff\" -> 0.000000000000   ,  \"Imoff\" -> 0.000000000000   ,  \"στ1\" -> 0.000000000000   ,  \"στS\" -> 0.000000000000   ,  \"στN\" -> 0.000000000000    |>   , \n\"IDS0599_220609_RAW_cal__ref_\" ->   <|    \"ζ\" -> 0.172195485890   ,  \"τ1\" -> 0.041384778581   ,  \"τS\" -> 0.038526635798   ,  \"τN\" -> 0.004361184391   ,  \"τC\" -> 0.000785294253   ,  \"κ0\" -> 0.000000001211   ,  \"mm1\" -> 0.000113668710   ,  \"mm2\" -> 0.030854392047   ,  \"mm3\" -> 0.061474921303   ,  \"T\" -> 0.250000000000   ,  \"B\" -> 4.000000000000   ,  \"θ\" -> 90.000000000000   ,  \"Reoff\" -> -31567346.938775509600   ,  \"Imoff\" -> 0.000000000000   ,  \"στ1\" -> 0.007771542596   ,  \"στS\" -> 0.000527239898   ,  \"στN\" -> 0.000989287072    |>   , \n\"IDS0599_220609_RAW_cal__sam_\" ->   <|    \"ζ\" -> 0.000000000000   ,  \"τ1\" -> 0.000000000000   ,  \"τS\" -> 0.000000000000   ,  \"τN\" -> 0.000000000000   ,  \"τC\" -> 0.000000000000   ,  \"κ0\" -> 0.000000000000   ,  \"mm1\" -> 0.000000000000   ,  \"mm2\" -> 0.000000000000   ,  \"mm3\" -> 0.000000000000   ,  \"T\" -> 0.250000000000   ,  \"B\" -> 4.000000000000   ,  \"θ\" -> 90.000000000000   ,  \"Reoff\" -> 0.000000000000   ,  \"Imoff\" -> 0.000000000000   ,  \"στ1\" -> 0.000000000000   ,  \"στS\" -> 0.000000000000   ,  \"στN\" -> 0.000000000000    |>   , \n\"IDS0601_220609_RAW_cal__ref_\" ->   <|    \"ζ\" -> 0.088588946696   ,  \"τ1\" -> 0.041065464736   ,  \"τS\" -> 0.032932718499   ,  \"τN\" -> 0.001668080480   ,  \"τC\" -> 0.000981218773   ,  \"κ0\" -> 0.000000001942   ,  \"mm1\" -> 0.000077888432   ,  \"mm2\" -> 0.031092575692   ,  \"mm3\" -> 0.048542266701   ,  \"T\" -> 0.360000000000   ,  \"B\" -> 4.000000000000   ,  \"θ\" -> 90.000000000000   ,  \"Reoff\" -> -11367346.938775509600   ,  \"Imoff\" -> 0.000000000000   ,  \"στ1\" -> 0.003759438303   ,  \"στS\" -> 0.000267670309   ,  \"στN\" -> 0.000061047491    |>   , \n\"IDS0601_220609_RAW_cal__sam_\" ->   <|    \"ζ\" -> 0.000000000000   ,  \"τ1\" -> 0.000000000000   ,  \"τS\" -> 0.000000000000   ,  \"τN\" -> 0.000000000000   ,  \"τC\" -> 0.000000000000   ,  \"κ0\" -> 0.000000000000   ,  \"mm1\" -> 0.000000000000   ,  \"mm2\" -> 0.000000000000   ,  \"mm3\" -> 0.000000000000   ,  \"T\" -> 0.360000000000   ,  \"B\" -> 4.000000000000   ,  \"θ\" -> 90.000000000000   ,  \"Reoff\" -> 0.000000000000   ,  \"Imoff\" -> 0.000000000000   ,  \"στ1\" -> 0.000000000000   ,  \"στS\" -> 0.000000000000   ,  \"στN\" -> 0.000000000000    |>   , \n\"IDS0602_220609_RAW_cal__ref_\" ->   <|    \"ζ\" -> 0.070839718876   ,  \"τ1\" -> 0.038371041474   ,  \"τS\" -> 0.031637984426   ,  \"τN\" -> 0.001186889357   ,  \"τC\" -> 0.001025755146   ,  \"κ0\" -> 0.000000002344   ,  \"mm1\" -> 0.000065987726   ,  \"mm2\" -> 0.030166305884   ,  \"mm3\" -> 0.044314681623   ,  \"T\" -> 0.420000000000   ,  \"B\" -> 4.000000000000   ,  \"θ\" -> 90.000000000000   ,  \"Reoff\" -> -8473469.387755101550   ,  \"Imoff\" -> 0.000000000000   ,  \"στ1\" -> 0.001572734023   ,  \"στS\" -> 0.000244025601   ,  \"στN\" -> 0.000010717849    |>   , \n\"IDS0602_220609_RAW_cal__sam_\" ->   <|    \"ζ\" -> 0.000000000000   ,  \"τ1\" -> 0.000000000000   ,  \"τS\" -> 0.000000000000   ,  \"τN\" -> 0.000000000000   ,  \"τC\" -> 0.000000000000   ,  \"κ0\" -> 0.000000000000   ,  \"mm1\" -> 0.000000000000   ,  \"mm2\" -> 0.000000000000   ,  \"mm3\" -> 0.000000000000   ,  \"T\" -> 0.420000000000   ,  \"B\" -> 4.000000000000   ,  \"θ\" -> 90.000000000000   ,  \"Reoff\" -> 0.000000000000   ,  \"Imoff\" -> 0.000000000000   ,  \"στ1\" -> 0.000000000000   ,  \"στS\" -> 0.000000000000   ,  \"στN\" -> 0.000000000000    |>   , \n\"IDS0603_220609_RAW_cal__ref_\" ->   <|    \"ζ\" -> 0.046492492626   ,  \"τ1\" -> 0.038232445790   ,  \"τS\" -> 0.031093656328   ,  \"τN\" -> 0.000672520001   ,  \"τC\" -> 0.001537595786   ,  \"κ0\" -> 0.000000003028   ,  \"mm1\" -> 0.000065353683   ,  \"mm2\" -> 0.030996834866   ,  \"mm3\" -> 0.041950918075   ,  \"T\" -> 0.520000000000   ,  \"B\" -> 4.000000000000   ,  \"θ\" -> 90.000000000000   ,  \"Reoff\" -> -3085714.285714285450   ,  \"Imoff\" -> 0.000000000000   ,  \"στ1\" -> 0.001914222591   ,  \"στS\" -> 0.000173880223   ,  \"στN\" -> 0.000009749430    |>   , \n\"IDS0603_220609_RAW_cal__sam_\" ->   <|    \"ζ\" -> 0.000000000000   ,  \"τ1\" -> 0.000000000000   ,  \"τS\" -> 0.000000000000   ,  \"τN\" -> 0.000000000000   ,  \"τC\" -> 0.000000000000   ,  \"κ0\" -> 0.000000000000   ,  \"mm1\" -> 0.000000000000   ,  \"mm2\" -> 0.000000000000   ,  \"mm3\" -> 0.000000000000   ,  \"T\" -> 0.520000000000   ,  \"B\" -> 4.000000000000   ,  \"θ\" -> 90.000000000000   ,  \"Reoff\" -> 0.000000000000   ,  \"Imoff\" -> 0.000000000000   ,  \"στ1\" -> 0.000000000000   ,  \"στS\" -> 0.000000000000   ,  \"στN\" -> 0.000000000000    |>   , \n\"IDS0604_220609_RAW_cal__ref_\" ->   <|    \"ζ\" -> 0.038076441388   ,  \"τ1\" -> 0.037827631760   ,  \"τS\" -> 0.031677046924   ,  \"τN\" -> 0.000456015371   ,  \"τC\" -> 0.001552950065   ,  \"κ0\" -> 0.000000003729   ,  \"mm1\" -> 0.000054479261   ,  \"mm2\" -> 0.031856398472   ,  \"mm3\" -> 0.040826279050   ,  \"T\" -> 0.620000000000   ,  \"B\" -> 4.000000000000   ,  \"θ\" -> 90.000000000000   ,  \"Reoff\" -> -2502040.816326530650   ,  \"Imoff\" -> 0.000000000000   ,  \"στ1\" -> 0.001808471812   ,  \"στS\" -> 0.000207619665   ,  \"στN\" -> 0.000014710860    |>   , \n\"IDS0604_220609_RAW_cal__sam_\" ->   <|    \"ζ\" -> 0.000000000000   ,  \"τ1\" -> 0.000000000000   ,  \"τS\" -> 0.000000000000   ,  \"τN\" -> 0.000000000000   ,  \"τC\" -> 0.000000000000   ,  \"κ0\" -> 0.000000000000   ,  \"mm1\" -> 0.000000000000   ,  \"mm2\" -> 0.000000000000   ,  \"mm3\" -> 0.000000000000   ,  \"T\" -> 0.620000000000   ,  \"B\" -> 4.000000000000   ,  \"θ\" -> 90.000000000000   ,  \"Reoff\" -> 0.000000000000   ,  \"Imoff\" -> 0.000000000000   ,  \"στ1\" -> 0.000000000000   ,  \"στS\" -> 0.000000000000   ,  \"στN\" -> 0.000000000000    |>   , \n\"IDS0605_220609_RAW_cal__ref_\" ->   <|    \"ζ\" -> 0.029084199331   ,  \"τ1\" -> 0.037802339111   ,  \"τS\" -> 0.034441444992   ,  \"τN\" -> 0.000221453940   ,  \"τC\" -> 0.001674221350   ,  \"κ0\" -> 0.000000005054   ,  \"mm1\" -> 0.000045238028   ,  \"mm2\" -> 0.034605412143   ,  \"mm3\" -> 0.040496951884   ,  \"T\" -> 0.820000000000   ,  \"B\" -> 4.000000000000   ,  \"θ\" -> 90.000000000000   ,  \"Reoff\" -> -1648979.591836734680   ,  \"Imoff\" -> 0.000000000000   ,  \"στ1\" -> 0.004366885644   ,  \"στS\" -> 0.000226589736   ,  \"στN\" -> 0.000007619141    |>   , \n\"IDS0605_220609_RAW_cal__sam_\" ->   <|    \"ζ\" -> 0.000000000000   ,  \"τ1\" -> 0.000000000000   ,  \"τS\" -> 0.000000000000   ,  \"τN\" -> 0.000000000000   ,  \"τC\" -> 0.000000000000   ,  \"κ0\" -> 0.000000000000   ,  \"mm1\" -> 0.000000000000   ,  \"mm2\" -> 0.000000000000   ,  \"mm3\" -> 0.000000000000   ,  \"T\" -> 0.820000000000   ,  \"B\" -> 4.000000000000   ,  \"θ\" -> 90.000000000000   ,  \"Reoff\" -> 0.000000000000   ,  \"Imoff\" -> 0.000000000000   ,  \"στ1\" -> 0.000000000000   ,  \"στS\" -> 0.000000000000   ,  \"στN\" -> 0.000000000000    |>   , \n\"IDS0606_220609_RAW_cal__ref_\" ->   <|    \"ζ\" -> 0.021888227668   ,  \"τ1\" -> 0.037829739612   ,  \"τS\" -> 0.039149374988   ,  \"τN\" -> 0.000098261842   ,  \"τC\" -> 0.001756976577   ,  \"κ0\" -> 0.000000007009   ,  \"mm1\" -> 0.000036081312   ,  \"mm2\" -> 0.037036868509   ,  \"mm3\" -> 0.042620464409   ,  \"T\" -> 1.100000000000   ,  \"B\" -> 4.000000000000   ,  \"θ\" -> 90.000000000000   ,  \"Reoff\" -> -840816.326530613004   ,  \"Imoff\" -> 0.000000000000   ,  \"στ1\" -> 0.002337246267   ,  \"στS\" -> 0.000239648135   ,  \"στN\" -> 0.000002696186    |>   , \n\"IDS0606_220609_RAW_cal__sam_\" ->   <|    \"ζ\" -> 0.000000000000   ,  \"τ1\" -> 0.000000000000   ,  \"τS\" -> 0.000000000000   ,  \"τN\" -> 0.000000000000   ,  \"τC\" -> 0.000000000000   ,  \"κ0\" -> 0.000000000000   ,  \"mm1\" -> 0.000000000000   ,  \"mm2\" -> 0.000000000000   ,  \"mm3\" -> 0.000000000000   ,  \"T\" -> 1.100000000000   ,  \"B\" -> 4.000000000000   ,  \"θ\" -> 90.000000000000   ,  \"Reoff\" -> 0.000000000000   ,  \"Imoff\" -> 0.000000000000   ,  \"στ1\" -> 0.000000000000   ,  \"στS\" -> 0.000000000000   ,  \"στN\" -> 0.000000000000    |>   , \n\"IDS0607_220609_RAW_cal__ref_\" ->   <|    \"ζ\" -> 0.018621761780   ,  \"τ1\" -> 0.037381709477   ,  \"τS\" -> 0.015442772270   ,  \"τN\" -> 0.000037477448   ,  \"τC\" -> 0.001928945161   ,  \"κ0\" -> 0.000000010412   ,  \"mm1\" -> 0.000031467858   ,  \"mm2\" -> 0.017593885804   ,  \"mm3\" -> 0.037453820216   ,  \"T\" -> 1.600000000000   ,  \"B\" -> 4.000000000000   ,  \"θ\" -> 90.000000000000   ,  \"Reoff\" -> -583673.469387755030   ,  \"Imoff\" -> 0.000000000000   ,  \"στ1\" -> 0.004296807814   ,  \"στS\" -> 0.000140639084   ,  \"στN\" -> 0.000001749476    |>   , \n\"IDS0607_220609_RAW_cal__sam_\" ->   <|    \"ζ\" -> 0.000000000000   ,  \"τ1\" -> 0.000000000000   ,  \"τS\" -> 0.000000000000   ,  \"τN\" -> 0.000000000000   ,  \"τC\" -> 0.000000000000   ,  \"κ0\" -> 0.000000000000   ,  \"mm1\" -> 0.000000000000   ,  \"mm2\" -> 0.000000000000   ,  \"mm3\" -> 0.000000000000   ,  \"T\" -> 1.600000000000   ,  \"B\" -> 4.000000000000   ,  \"θ\" -> 90.000000000000   ,  \"Reoff\" -> 0.000000000000   ,  \"Imoff\" -> 0.000000000000   ,  \"στ1\" -> 0.000000000000   ,  \"στS\" -> 0.000000000000   ,  \"στN\" -> 0.000000000000    |>   , \n\"IDS0608_220610_RAW_cal__ref_\" ->   <|    \"ζ\" -> 0.016544796602   ,  \"τ1\" -> 0.037383789571   ,  \"τS\" -> 0.013791768179   ,  \"τN\" -> 0.000022452051   ,  \"τC\" -> 0.002003011160   ,  \"κ0\" -> 0.000000012629   ,  \"mm1\" -> 0.000028575716   ,  \"mm2\" -> 0.015977354879   ,  \"mm3\" -> 0.037423643830   ,  \"T\" -> 1.900000000000   ,  \"B\" -> 4.000000000000   ,  \"θ\" -> 90.000000000000   ,  \"Reoff\" -> -306122.448979591834   ,  \"Imoff\" -> 0.000000000000   ,  \"στ1\" -> 0.018453773805   ,  \"στS\" -> 0.003656712594   ,  \"στN\" -> 0.000009862061    |>   , \n\"IDS0608_220610_RAW_cal__sam_\" ->   <|    \"ζ\" -> 0.000000000000   ,  \"τ1\" -> 0.000000000000   ,  \"τS\" -> 0.000000000000   ,  \"τN\" -> 0.000000000000   ,  \"τC\" -> 0.000000000000   ,  \"κ0\" -> 0.000000000000   ,  \"mm1\" -> 0.000000000000   ,  \"mm2\" -> 0.000000000000   ,  \"mm3\" -> 0.000000000000   ,  \"T\" -> 1.900000000000   ,  \"B\" -> 4.000000000000   ,  \"θ\" -> 90.000000000000   ,  \"Reoff\" -> 0.000000000000   ,  \"Imoff\" -> 0.000000000000   ,  \"στ1\" -> 0.000000000000   ,  \"στS\" -> 0.000000000000   ,  \"στN\" -> 0.000000000000    |>   , \n\"IDS0609_220610_RAW_cal__ref_\" ->   <|    \"ζ\" -> 0.016105107000   ,  \"τ1\" -> 0.037302695889   ,  \"τS\" -> 0.009839075109   ,  \"τN\" -> 0.000006613992
